vi "Apply styles to GObjects.vi"(8 "Error In":errorcluster, 10 "Style Sheet":string, 11 "Front Panel Objects":refnum<vi>[](array[refnum])) -> (0 "Error Out":errorcluster, 3 "Front Panel Objects (dup)":refnum<vi>[](array[refnum]))   [LabVIEW 2019, in "LSS.lvlib"]
doc: "Parses the text from the style sheet input to find relevent properties which apply to the each front panel object input, then applies these properties to all controls.\n\n<b>Inputs:</b>\n<b>Front Panel Object</b> - All Front panel objects that can be modified by LabVIEW programatically.\n<b>Style Sheet</b> - Text style sheet which will be applied to the front panel element.\n<b>Error In</b> - Error input terminal.\n\n<b>Outputs:</b>\n<b>Front Panel Object (dup) </b> - All front panel objects duplicated on the output terminal for easier diagram layout.\n<b>Error Out</b> - Error output terminal."
uses:
  LSS.lvlib
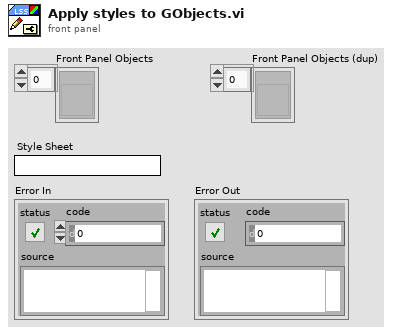
[diagram p1: front panel]
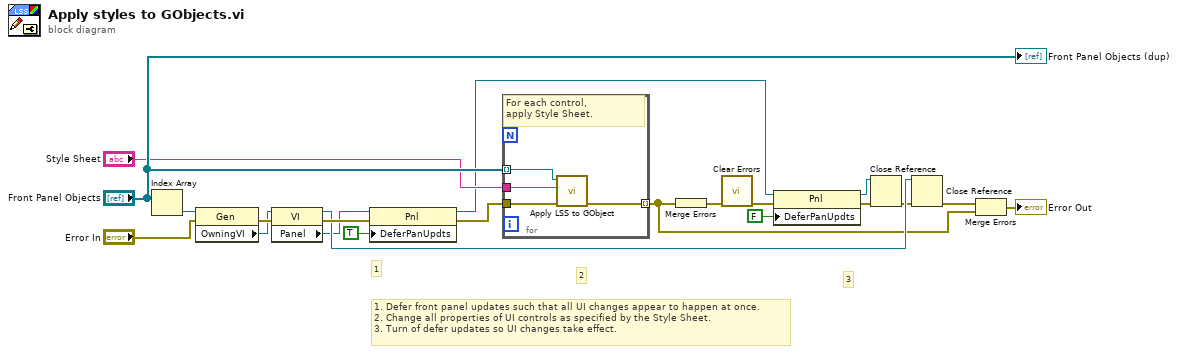
[diagram p0: block diagram]
diagram:
  # "1. Defer front panel updates such that all UI changes appear to happen at once.\n2. Change all properties of UI controls as specified by the Style Sheet.\n3. Turn of defer updates so UI changes take effect."
  # "3"
  # "2"
  # "1"
  n1 = Index Array(array="Front Panel Objects") -> (element=w14:refnum<vi>)  [unwired: 1 in]
  n2 = property class="Gen"(reference=w14, error in="Error In") -> (error out=w21:errorcluster, "OwningVI"=w15:refnum<vi>)  [unwired: 1 out]
  n3 = property class="VI"(reference=w15, error in=w21) -> (reference out=w19:refnum<vi>, error out=w20:errorcluster, "Panel"=w9:refnum<vi>)
  n4 = property class="Pnl"(reference=w9, error in=w20, "DeferPanUpdts"=TRUE ("Defer Panel Updates")) -> (reference out=w4:refnum<vi>, error out=w11:errorcluster)
  n5 = for {
    tunnel: "Style Sheet" -> [w25]
    tunnel: "Front Panel Objects" -> [w24] mode=indexing
    tunnel: w11 -> [w23]
    tunnel: [w22] -> w3 mode=indexing
    # "For each control,\napply Style Sheet."
    n6 = call "Apply LSS to GObject.vi"("Error in"=w23, "Style Sheet"=w25, "Gen Refnum"=w24) -> ("Error out"=w22:errorcluster)  [unwired: 8 in]
  }
  n7 = Merge Errors(w3) -> (w2:errorcluster)
  n8 = call <vilib>:"Clear Errors.vi"("error in (no error)"=w2) -> ("error out"=w1:errorcluster)  [unwired: 5 in, 1 out]
  n9 = property class="Pnl"(reference=w4, error in=w1, "DeferPanUpdts"=FALSE ("Defer Panel Updates")) -> (reference out=w17:refnum<vi>, error out=w16:errorcluster)
  n10 = Close Reference(reference=w17, error in (no error)=w16) -> (error out=w18:errorcluster)
  n11 = Close Reference(reference=w19, error in (no error)=w18) -> (error out=w7:errorcluster)
  n12 = Merge Errors(w7, w3) -> (→"Error Out":errorcluster)
  "Front Panel Objects (dup)" <- "Front Panel Objects"
